vi "Constants.vi"() -> ()   [LabVIEW 2020, in "Ballard ARINC 429 Hardware Configuration.lvlib"]
uses:
  Ballard ARINC 429 Hardware Configuration.lvlib
panel:
  in  "zzzTab":enum32{"Core", "Rx", "Tx", "Label"}(tab)
  in  "Core.Format":string="<bti:core xmlns:bti=\"http://www.ballardtech.com/DatabusSchemas/\" xmlns:xs=\"http://www.w3.org/2001/XMLSchema-instance\" ID=\"0\" name=\"Core_%d\" schemaVersion=\"1.0\">\n\t<bti:coreConfiguration>\n\t\t<bti:sequentialLog perChannelStreaming=\"false\"/>\n\t\t<bti:builtInTest/>\n\t\t<bti:pxi/>\n\t\t<bti:sysMon/>\n\t\t<bti:timing/>\n\t</bti:coreConfiguration>\n"
  in  "Core.Final":string="\n</bti:core>\n"
  in  "Rx.Channel":string="\t<bti:channel429 ID=\"%d\" name=\"CH%d\" hardwareChannel=\"%d\" monitorMode=\"Selective\">\n\t\t<bti:rxChannel speedKHz=\"100\">\n"
  in  "Rx.Channel End":string="\t\t\t</bti:labels>\n\t\t</bti:rxChannel>\n\t</bti:channel429>\n"
  in  "Rx.Header":string="\n<!--***************************************\tRx Channels ***************************************-->\n"
  in  "Tx.Scheduled Buffer SDI":string="\t\t\t\t\t<bti:messageBuffers>\n\t\t\t\t\t\t<bti:messageBuffer ID=\"%d\" name=\"MessageBuffer_label %d_%d\">\n\t\t\t\t\t\t\t<bti:rawData>%s</bti:rawData>\n\t\t\t\t\t\t</bti:messageBuffer>\n\t\t\t\t\t</bti:messageBuffers>\n\t\t\t\t</bti:message>\n"
  in  "Tx.Scheduled Message Info SDI":string="\t\t\t\t<bti:message ID=\"%d\" name=\"label %d_%d\" messageBufferIDRef=\"%d\" minRate=\"10\" maxRate=\"10\" labelDecimal=\"%d\" SDI=\"%02b\">\n"
  in  "Tx.Acyclic Buffer List End":string="\t\t\t\t</bti:messageBuffers>\n"
  in  "Tx.Acyclic Buffer List Start":string="\t\t\t\t<bti:messageBuffers>\n"
  in  "Tx.Scheduled Message Info":string="\t\t\t\t<bti:message ID=\"%d\" name=\"label %d\" messageBufferIDRef=\"%d\" minRate=\"10\" maxRate=\"10\" labelDecimal=\"%d\">\n"
  in  "Tx.Header":string="\n<!--***************************************\tTx Channels ***************************************-->\n"
  in  "Tx.Channel":string="\t<bti:channel429 ID=\"%d\" name=\"CH%d\" hardwareChannel=\"%d\">\n\t\t<bti:txChannel speedKHz=\"100\" scheduleMode=\"Rate\" highVolt=\"10\" lowVolt=\"-10\" nullVolt=\"0\" cmBiasVolt=\"0\" highRiseTime=\"1.8\" lowRiseTime=\"1.8\">\n"
  in  "Tx.Channel End":string="\t\t</bti:txChannel>\n\t</bti:channel429>\n"
  in  "Tx.Acyclic Message List":string="\t\t\t<bti:asyncMessageList>\n"
  in  "Tx.Acyclic Message List End":string="\t\t\t</bti:asyncMessageList>\n"
  in  "Tx.Acyclic Buffer":string="\t\t\t\t\t<bti:messageBuffer ID=\"%d\" name=\"Acyclic %03d\">\n\t\t\t\t\t\t<bti:rawData>%s</bti:rawData>\n\t\t\t\t\t</bti:messageBuffer>\n"
  in  "Tx.Scheduled Messages":string="\t\t\t<bti:messages>\n"
  in  "Tx.Scheduled Buffer":string="\t\t\t\t\t<bti:messageBuffers>\n\t\t\t\t\t\t<bti:messageBuffer ID=\"%d\" name=\"MessageBuffer_label %d\">\n\t\t\t\t\t\t\t<bti:rawData>%s</bti:rawData>\n\t\t\t\t\t\t</bti:messageBuffer>\n\t\t\t\t\t</bti:messageBuffers>\n\t\t\t\t</bti:message>\n"
  in  "Tx.Scheduled Messages End":string="\t\t\t</bti:messages>\n"
  in  "Label.Begin":string="\t\t\t<bti:labels>\n"
  in  "Label.Info":string="\t\t\t\t<bti:label ID=\"%d\" name=\"label %d\" labelDecimal=\"%d\" monitor=\"true\"/>\n"
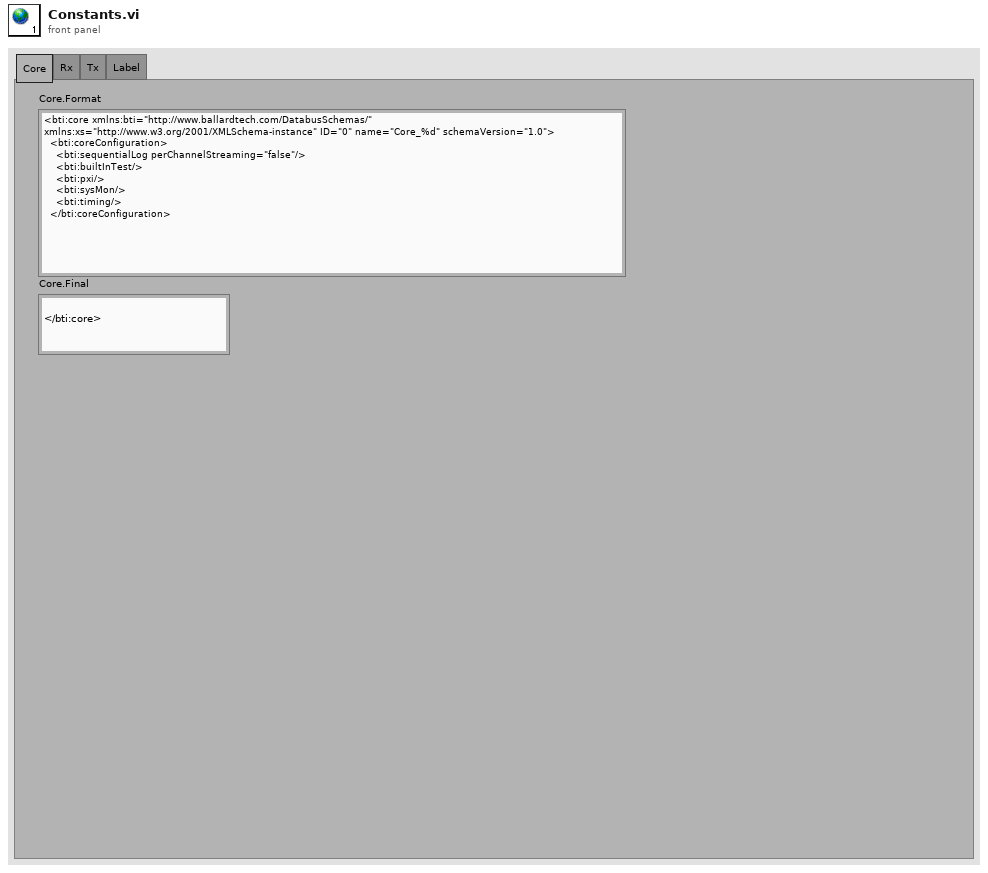
[diagram p1: front panel]
diagram:
